vi "DMLSFM_PULSE_REDUCER_FOR_OPTIMISATION.vi"() -> ()   [LabVIEW 2017]
doc: "This example demonstrates how to generate a finite amount of digital data based off of a sample clock.\n\nSome hardware (e.g. M Series DAQ) must use an external sample clock for digital tasks. To view a complete list of available sample clock sources, consult the Device Routes table in Measurement and Automation Explorer.\n\nFor instructions on how to connect your signals to the DAQ device, refer to your device documentation."
uses:
  <vilib>/Utility/error.llb/DialogType.ctl
  <vilib>/DAQmx/write.llb/DAQmx Write (Digital 1D U32 1Chan NSamp).vi
  <vilib>/DAQmx/create/channels.llb/DAQmx Create Channel (DO-Digital Output).vi
  <vilib>/DAQmx/configure/timing.llb/DAQmx Timing (Sample Clock).vi
  <vilib>/DAQmx/configure/trigger.llb/DAQmx Start Trigger (Digital Edge).vi
  <vilib>/DAQmx/miscellaneous.llb/DAQmx Fill In Error Info.vi
  <resource>/objmgr/daqmx.rc
panel:
  out "error out":errorcluster
  in  "stop":bool
  in  "Output Array":u32[](array[numeric])=[1, 1, 1, 1, 1, 1, 0, 0, 0, 0, 0, 0, 0, 0, 0, 0, 0, 0, 0, 0, 0]
  in  "Trigger Type":enum32{"No Trigger", "Digital Start"}(tab)=enum."Digital Start"
  in  "Edge":i32(ring)=10280 items=["Rising"=10280, "Falling"=10171]
  in  "Digital Trigger Source":tag="PFI1"
  in  "Number of Samples":i32=10
  in  "Sample Rate":dbl=10000.0
  in  "Sample Clock Source":tag="OnboardClock"
  out "Actual Sample Rate":dbl=100000.0 format="%0.2f"
  in  "Line(s)":tag="Dev4/port0/line0"
  # "Channel Settings"
  # "Data to Write"
  # "Timing and Buffer Settings"
  # "Trigger Settings"
  # "To configure and use a start trigger you must have the necessary tab selected above.  Not all hardware supports triggering--refer to your device documentation for more info."
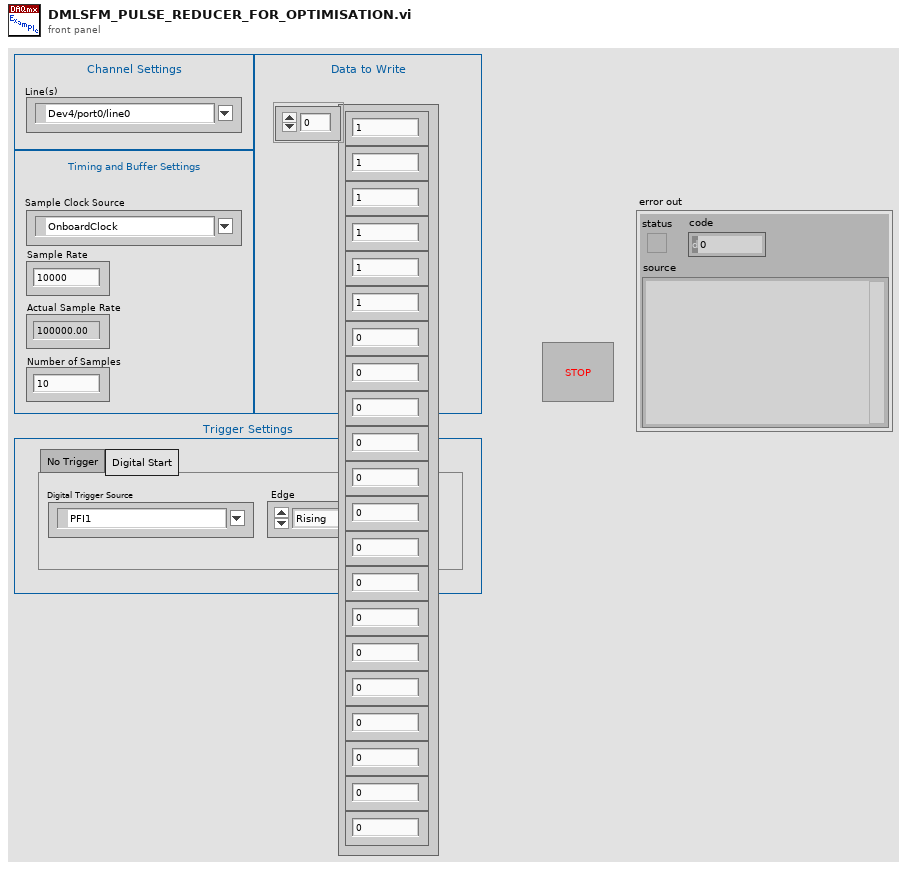
[diagram p1: front panel]
types:
  T1 = typedef "DialogType.ctl" = u16
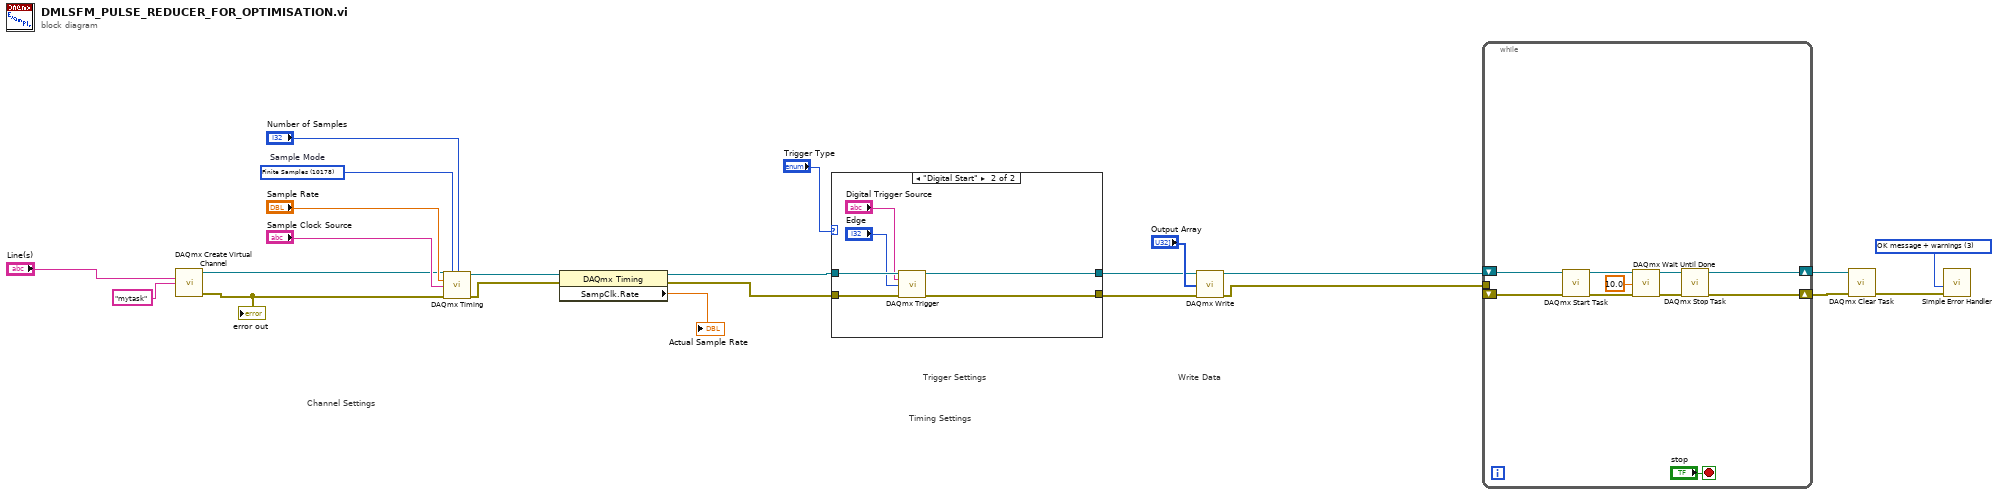
[diagram p0: block diagram]
diagram:
  w11 = T1 3 items=["no dialog", "OK message", "continue or stop message", "OK message + warnings", "continue/stop + warnings"] ("type of dialog (OK msg:1)")
  w13 = 10178 items=["Finite Samples"=10178, "Continuous Samples"=10123, "Hardware Timed Single Point"=12522]  # Sample Mode
  # "Trigger Settings"
  # "Timing Settings"
  # "Write Data"
  # "Channel Settings"
  n1 = call-poly <vilib>:"DAQmx Create Virtual Channel.vi"("lines"="Line(s)", "name to assign"="mytask") -> ("task out"=w1:refnum<k21>, "error out"=w12:errorcluster)  [unwired: 12 in]
  "error out" <- w12
  n2 = call-poly <vilib>:"DAQmx Timing.vi"("task/channels in"=w1, "sample mode"=w13, "samples per channel"="Number of Samples", "rate"="Sample Rate", "source"="Sample Clock Source", "error in"=w12) -> ("task out"=w17:refnum<k21>, "error out"=w18:errorcluster)  [unwired: 8 in]
  n3 = property class="DAQmx Timing"(reference=w17, error in=w18) -> (reference out=w6:refnum<k21>, error out=w5:errorcluster, "SampClk.Rate"=→"Actual Sample Rate":dbl)
  n4 = case shown="\"Digital Start\"" "Trigger Type" {
    tunnel: w6 -> [w25 w31]
    tunnel: w5 -> [w24 w30]
    tunnel: [w25 w29] -> w8
    tunnel: [w24 w28] -> w9
    frame "No Trigger", Default {
    }
    frame "Digital Start" {
      n5 = call-poly <vilib>:"DAQmx Trigger.vi"("task/channels in"=w31, "source"="Digital Trigger Source", "edge"="Edge", "error in"=w30) -> ("task out"=w29:refnum<k21>, "error out"=w28:errorcluster)  [unwired: 10 in]
    }
  }
  n6 = call-poly <vilib>:"DAQmx Write.vi"("task/channels in"=w8, "data"="Output Array", "error in"=w9) -> ("task out"=w3:refnum<k21>, "error out"=w4:errorcluster)  [unwired: 10 in, 1 out]
  n7 = while {
    shift-right: [w37] -> w22
    shift-left: w3 -> [w32]
    shift-right: [w36] -> w21
    shift-left: _ -> [_]
    tunnel: w4 -> [w33]
    stop <- "stop" stop-if-true
    n8 = call <vilib>:"DAQmx Start Task.vi"("task/channels in"=w32, "error in"=w33) -> ("task out"=w41:refnum<k21>, "error out"=w40:errorcluster)  [unwired: 12 in]
    n9 = call <vilib>:"DAQmx Wait Until Done.vi"("task/channels in"=w41, "timeout (sec)"=10.0, "error in"=w40) -> ("task out"=w39:refnum<k21>, "error out"=w38:errorcluster)  [unwired: 11 in]
    n10 = call <vilib>:"DAQmx Stop Task.vi"("task/channels in"=w39, "error in"=w38) -> ("task out"=w37:refnum<k21>, "error out"=w36:errorcluster)  [unwired: 12 in]
  }
  n11 = call <vilib>:"DAQmx Clear Task.vi"("task in"=w22, "error in"=w21) -> ("error out"=w23:errorcluster)  [unwired: 13 in]
  n12 = call <vilib>:"Simple Error Handler.vi"("type of dialog (OK msg:1)"=w11, "error in (no error)"=w23) -> ()  [unwired: 3 in, 5 out]
